vi "Read Measurement.vi"(8 "error in (no error)":errorcluster, 10 "Timeout (10000 ms)":u32=10000, 11 "VISA resource name":refnum<visa-resource-name>) -> (0 "error out":errorcluster, 2 "Measurement":dbl, 3 "VISA resource name out":refnum<visa-resource-name>)   [LabVIEW 2015, in "Template - Power Meter.lvlib"]
doc: "Performs a single, new measurement and outputs the result.\n\n<b>Note: </b>The type of measurement returned is determined by calling the <b>Configure Measurement</b> VI."
uses:
  <instrlib>/_Template - Power Meter/Template - Power Meter.lvlib
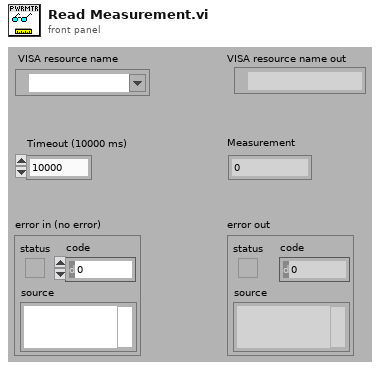
[diagram p1: front panel]
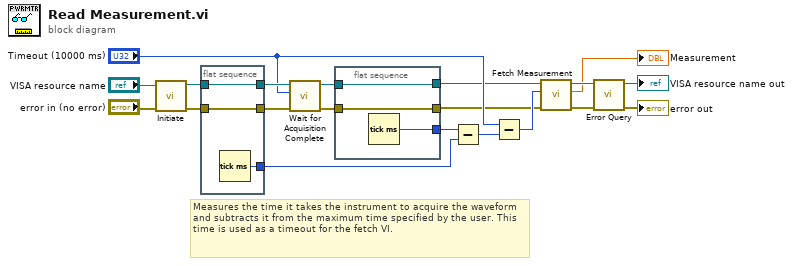
[diagram p0: block diagram]
diagram:
  # "Measures the time it takes the instrument to acquire the waveform and subtracts it from the maximum time specified by the user. This time is used as a timeout for the fetch VI."
  n1 = call <instrlib>:"Initiate.vi"("error in (no error)"="error in (no error)", "VISA resource name"="VISA resource name") -> ("error out"=w10:errorcluster, "VISA resource name out"=w11:refnum<visa-resource-name>)  [unwired: 8 in]
  n2 = flat-sequence {
    tunnel: [w23] -> w7
    tunnel: w11 -> [w23]
    tunnel: [w22] -> w8
    tunnel: w10 -> [w22]
    tunnel: [w21] -> w9
    frame #0 {
      n3 = Tick Count (ms)() -> (millisecond timer value=w21:u32)
    }
  }
  n4 = call <instrlib>:"Wait for Acquisition Complete.vi"("error in (no error)"=w8, "Maximum Time (10000 ms)"="Timeout (10000 ms)", "VISA resource name"=w7) -> ("error out"=w4:errorcluster, "VISA resource name out"=w5:refnum<visa-resource-name>)  [unwired: 7 in]
  n5 = flat-sequence {
    tunnel: [w26] -> w2
    tunnel: w5 -> [w26]
    tunnel: [w25] -> w1
    tunnel: w4 -> [w25]
    tunnel: [w24] -> w3
    frame #0 {
      n6 = Tick Count (ms)() -> (millisecond timer value=w24:u32)
    }
  }
  n7 = Subtract(x=w3, y=w9) -> (x-y=w16:u32)
  n8 = Subtract(x="Timeout (10000 ms)", y=w16) -> (x-y=w12:u32)
  n9 = call <instrlib>:"Fetch Measurement.vi"("error in (no error)"=w1, "Timeout (10000 ms)"=w12, "VISA resource name"=w2) -> ("error out"=w14:errorcluster, "Measurement"=→"Measurement":dbl, "VISA resource name out"=w15:refnum<visa-resource-name>)  [unwired: 6 in]
  n10 = call <instrlib>:"Error Query.vi"("error in (no error)"=w14, "VISA resource name"=w15) -> ("error out"=→"error out":errorcluster, "VISA resource name out"=→"VISA resource name out":refnum<visa-resource-name>)  [unwired: 6 in, 2 out]
